vi "ReadAll.vi"(8 "error in (no error)":errorcluster, 11 "NetworkStreamReader in":refnum<class "NetworkStreamReader.lvclass">) -> (0 "error out":errorcluster, 1 "New element?":bool, 2 "elements":variant[](array[variant]), 3 "NetworkStreamReader out":refnum<class "NetworkStreamReader.lvclass">, 4 "Latest time stamp":timestamp)   [LabVIEW 2011, in "NetworkStreamReader.lvclass"]
uses:
  NetworkStreamReader.lvclass
  NetworkStreamReader.lvclass/NetworkStreamReader.ctl
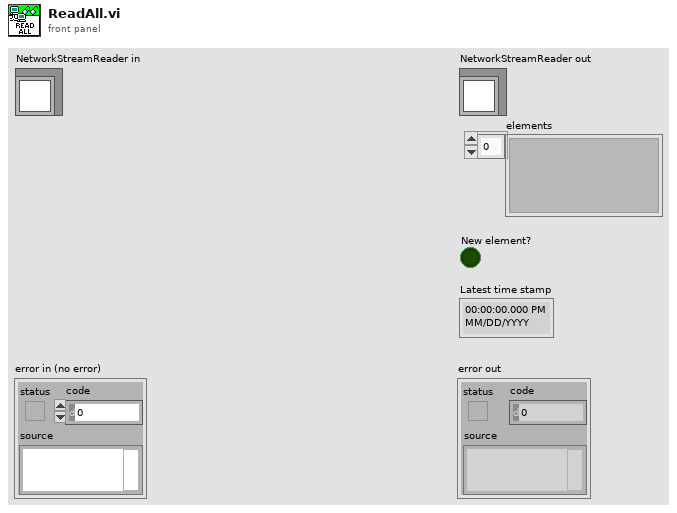
[diagram p1: front panel]
types:
  T1 = typedef "message.ctl" = cluster{"Data":variant, "Time since start (s)":dbl}
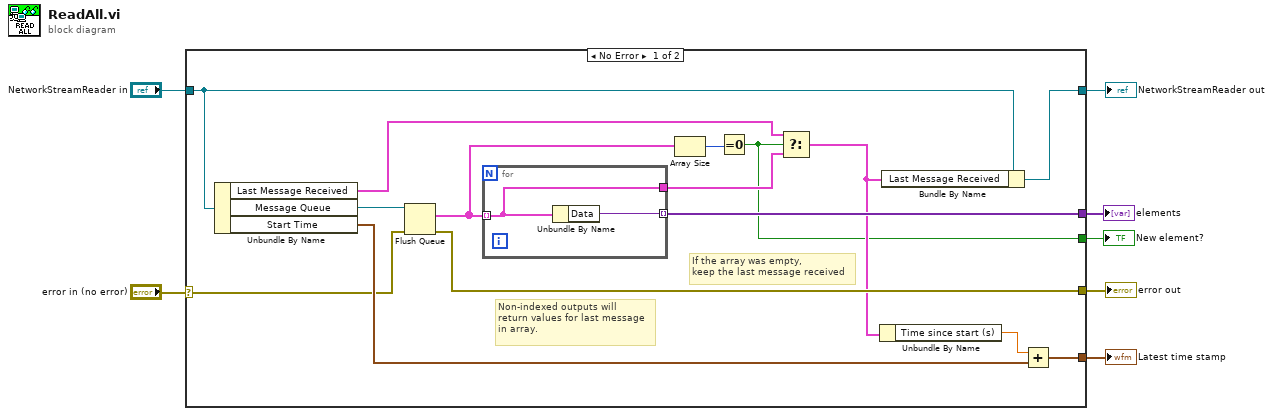
[diagram p0: block diagram]
diagram:
  n1 = case shown="No Error" "error in (no error)" {
    selector: "error in (no error)" -> [w18 w26]
    tunnel: [w16 w26] -> w6
    tunnel: [w21 w25] -> w5
    tunnel: "NetworkStreamReader in" -> [w22 w25]
    tunnel: [w17 _] -> w2
    tunnel: [w19 _] -> w3
    tunnel: [w8 _] -> w1
    frame No Error {
      # "If the array was empty,\nkeep the last message received"
      # "Non-indexed outputs will\nreturn values for last message\nin array."
      n2 = Unbundle By Name(w22) -> ("Last Message Received"=w12:T1, "Message Queue"=w13:refnum<queue>, "Start Time"=w20:timestamp)
      n3 = Flush Queue(queue=w13, error in (no error)=w18) -> (remaining elements=w15:T1[], error out=w16:errorcluster)  [unwired: 1 out]
      n4 = for {
        tunnel: w15 -> [w23] mode=indexing
        tunnel: [w24] -> w17 mode=indexing
        tunnel: [w23] -> w11
        n5 = Unbundle By Name(w23) -> ("Data"=w24:variant)
      }
      n6 = Array Size(array=w15) -> (size(s)=w14:i32)
      n7 = Equal To 0?(x=w14) -> (x = 0?=w8:bool)
      n8 = Select(t=w12, s=w8, f=w11) -> (s? t:f=w10:T1)
      n9 = Unbundle By Name(w10) -> ("Time since start (s)"=w9:dbl)
      n10 = Bundle By Name(cluster=w22, "Last Message Received"=w10) -> (w21:refnum<class "NetworkStreamReader.lvclass">)
      n11 = Add(x=w9, y=w20) -> (x+y=w19:timestamp)
    }
    frame Error {
    }
  }
  "error out" <- w6
  "NetworkStreamReader out" <- w5
  "Latest time stamp" <- w3
  "elements" <- w2
  "New element?" <- w1
